vi "Set trigger.vi"(8 "error in (no error)":errorcluster, 11 "StageSPIM in":refnum<class "StageSPIM.lvclass">) -> (0 "error out":errorcluster, 3 "StageSPIM out":refnum<class "StageSPIM.lvclass">)   [LabVIEW 2012, in "StageSPIM.lvclass"]
uses:
  StageSPIM.lvclass
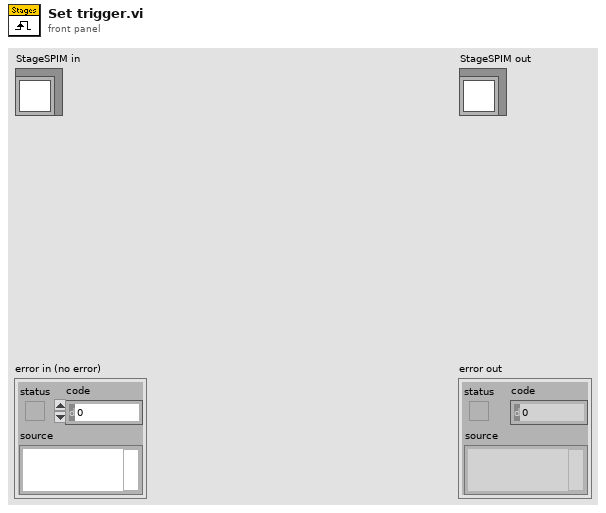
[diagram p1: front panel]
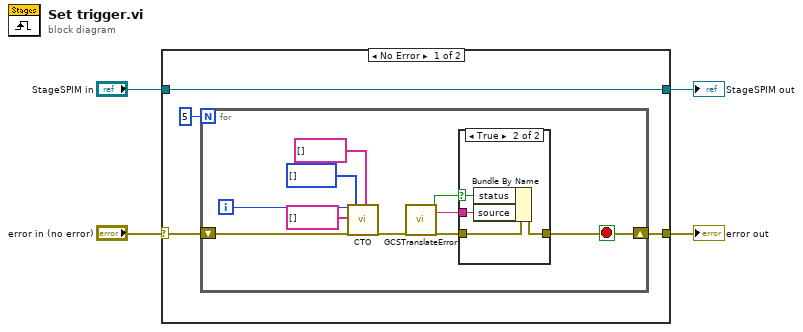
[diagram p0: block diagram]
diagram:
  n1 = case shown="No Error" "error in (no error)" {
    selector: "error in (no error)" -> [w6 w25]
    tunnel: [w5 w25] -> w3
    tunnel: [w8 w24] -> w1
    tunnel: "StageSPIM in" -> [w8 w24]
    frame No Error {
      n2 = for {
        N: 5 -> [_]
        shift-right: [w9] -> w5
        shift-left: w6 -> [w18]
        i -> [w17]
        stop <- w9 stop-if-true
        n3 = call "CTO.vi"("System no."=w17, "TriggerOut to set"=string[] [], "error in"=w18, "CTO parameter ID"=i32[] [], "Parameter value"=string[] []) -> ("error out"=w10:errorcluster)  [unwired: 13 in, 1 out]
        n4 = call "GCSTranslateError.vi"("error in"=w10) -> ("GCS Error?"=w12:bool, "Error Description"=w11:string, "error out"=w13:errorcluster)  [unwired: 16 in]
        n5 = case shown="True" w12 {
          selector: w12 -> [_ w21]
          tunnel: w13 -> [w19 w23]
          tunnel: [w19 w22] -> w9
          tunnel: w11 -> [_ w20]
          frame False {
          }
          frame True {
            n6 = Bundle By Name(cluster=w23, "status"=w21, "source"=w20) -> (w22:errorcluster)
          }
        }
      }
    }
    frame Error {
    }
  }
  "error out" <- w3
  "StageSPIM out" <- w1
